vi "Folder Check (SubVI).vi"(7 "System Message Queue In":refnum<queue>, 8 "error in (no error)":errorcluster) -> (0 "error out":errorcluster)   [LabVIEW 2019]
uses:
  Globals and Definitions/System Message.ctl
  Globals and Definitions/Initialization Globals.vi
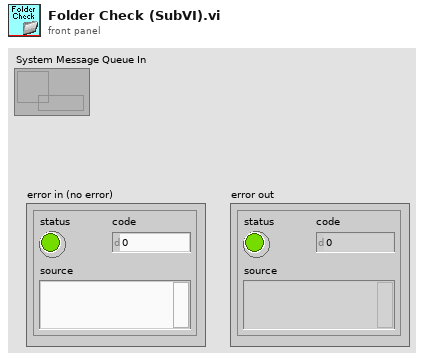
[diagram p1: front panel]
types:
  T1 = typedef "System Message.ctl" = cluster{"Message Tag":string, "Message Body":string, "Snooze Time (s)":dbl, "Snooze Alert?":bool, "Log Event?":bool, "Send Email":i32}
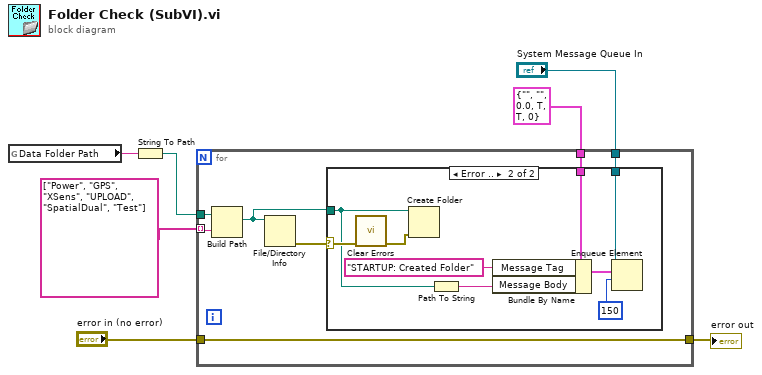
[diagram p0: block diagram]
diagram:
  n1 = global read "Initialization Globals.vi" "Data Folder Path"() -> (w6:string)
  n2 = String To Path(string=w6) -> (path=w5:path)
  n3 = for {
    tunnel: string[] ["Power", "GPS", "XSens", "UPLOAD", "SpatialDual", "Test"] -> [w12] mode=indexing
    tunnel: w5 -> [w11]
    tunnel: T1 {"Message Tag"="", "Message Body"="", "Snooze Time (s)"=0.0, "Snooze Alert?"=TRUE, "Log Event?"=TRUE, "Send Email"=0} -> [w10]
    tunnel: "System Message Queue In" -> [w9]
    tunnel: "error in (no error)" -> [w8]
    tunnel: [w8] -> w1
    n4 = Build Path(base path=w11, name or relative path=w12) -> (appended path=w14:path)
    n5 = File/Directory Info(path=w14) -> (error out=w13:errorcluster)  [unwired: 1 in, 6 out]
    n6 = case shown="Error .." w13 {
      selector: w13 -> [_ w23]
      tunnel: w14 -> [_ w16]
      tunnel: w10 -> [_ w19]
      tunnel: w9 -> [_ w18]
      frame No Error {
      }
      frame Error {
        n7 = call <vilib>:"Clear Errors.vi"("error in (no error)"=w23) -> ("error out"=w22:errorcluster)  [unwired: 5 in, 1 out]
        n8 = Create Folder(path (use dialog)=w16, error in=w22) -> ()  [unwired: 1 in, 3 out]
        n9 = Path To String(path=w16) -> (string=w15:string)
        n10 = Bundle By Name(cluster=w19, "Message Tag"="STARTUP: Created Folder", "Message Body"=w15) -> (w20:T1)
        n11 = Enqueue Element(queue=w18, element=w20, timeout in ms (-1)=150) -> ()  [unwired: 1 in, 3 out]
      }
    }
  }
  "error out" <- w1
